vi "Create vision based MM setpoints.vi"(1 "4Final distance away from the target to end":dbl format="%#_13g", 2 "Gyro":dbl, 3 "Vision's angle that the target is offcenter":dbl format="%#_13g", 4 "Vision's distance to target":dbl format="%#_13g") -> (0 "Vision-based MM Setpoints":T1(array[cluster]))   [LabVIEW 2018]
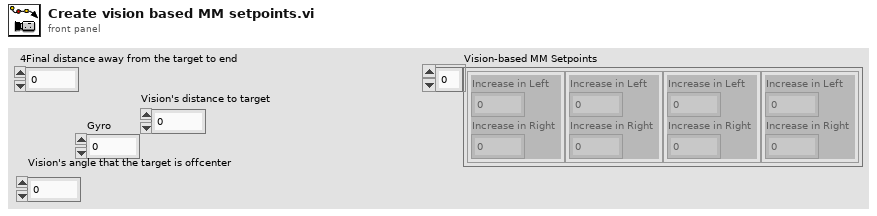
[diagram p1: front panel]
types:
  T1 = cluster{"Increase in Left":dbl, "Increase in Right":dbl}[]
  T2 = cluster{"Increase in Left":dbl, "Increase in Right":dbl}
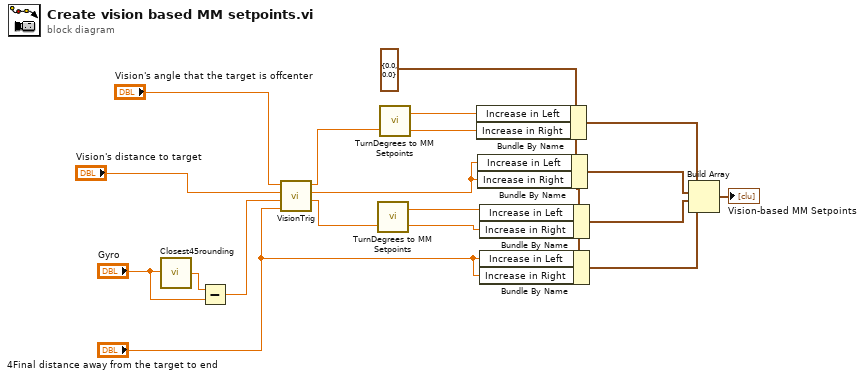
[diagram p0: block diagram]
diagram:
  w4 = T2 {"Increase in Left"=0.0, "Increase in Right"=0.0} ("Drive MM Setpoints")
  n1 = call "Closest45rounding.vi"("Gyro"="Gyro") -> ("Closest Angle"=w19:dbl)
  n2 = Subtract(x=w19, y="Gyro") -> (x-y=w17:dbl)
  n3 = call "VisionTrig.vi"("4Final distance away from the target to end"="4Final distance away from the target to end", "difference in heading between robot and target's perpindicular line"=w17, "Vision's distance to target"="Vision's distance to target", "Vision's angle that the target is offcenter"="Vision's angle that the target is offcenter") -> ("3Angle to turn to be perpindicular to the target"=w14:dbl, "2Distance to drive"=w10:dbl, "1 Angle to turn to get to the destination point"=w13:dbl)  [unwired: 5 in]
  n4 = call "TurnDegrees to MM Setpoints.vi"("Turn Degrees"=w14) -> ("Right MM Setpoint"=w8:dbl, "Left MM Setpoint"=w9:dbl)  [unwired: 1 in]
  n5 = call "TurnDegrees to MM Setpoints.vi"("Turn Degrees"=w13) -> ("Right MM Setpoint"=w11:dbl, "Left MM Setpoint"=w12:dbl)  [unwired: 1 in]
  n6 = Bundle By Name(cluster=w4, "Increase in Left"=w12, "Increase in Right"=w11) -> (w6:T2)
  n7 = Bundle By Name(cluster=w4, "Increase in Left"=w10, "Increase in Right"=w10) -> (w7:T2)
  n8 = Bundle By Name(cluster=w4, "Increase in Left"=w9, "Increase in Right"=w8) -> (w5:T2)
  n9 = Bundle By Name(cluster=w4, "Increase in Left"="4Final distance away from the target to end", "Increase in Right"="4Final distance away from the target to end") -> (w3:T2)
  n10 = Build Array(w6, w7, w5, w3) -> (→"Vision-based MM Setpoints":T1)
